vi "Utility Decode ID String.vi"(8 "error in (no error)":errorcluster, 10 "*IDN? Response":string, 11 "VISA resource name in":refnum<visa-resource-name>) -> (0 "error out":errorcluster, 2 "Unit Info":T1, 3 "VISA resource name out":refnum<visa-resource-name>)   [LabVIEW 2020, in "Berkeley Nucleonics 500 Series.lvlib"]
doc: "This VI decodes the response from an *IDN? query to return information about the unit It is private in scope."
uses:
  Berkeley Nucleonics 500 Series.lvlib
  Unit Info.ctl
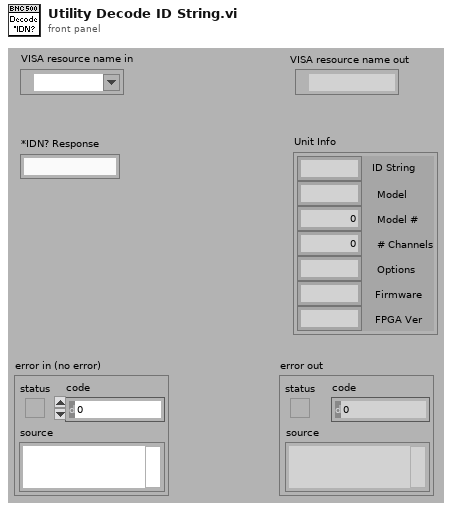
[diagram p1: front panel]
types:
  T1 = typedef "Berkeley Nucleonics 500 Series.lvlib/Unit Info.ctl" = cluster{"ID String":string, "Model":string, "Model #":i32, "# Channels":i32, "Options":string, "Firmware":string, "FPGA Ver":string}
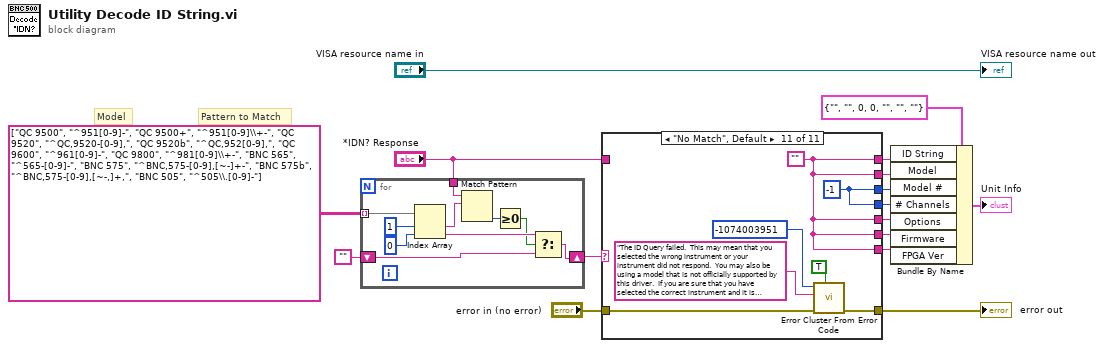
[diagram p0: block diagram]
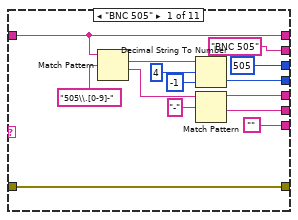
[diagram p2: hidden frame]
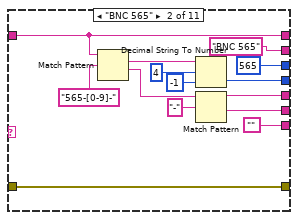
[diagram p3: hidden frame]
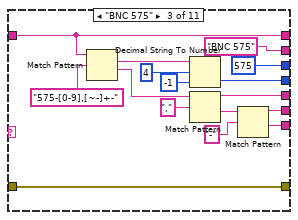
[diagram p4: hidden frame]
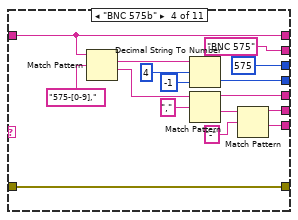
[diagram p5: hidden frame]
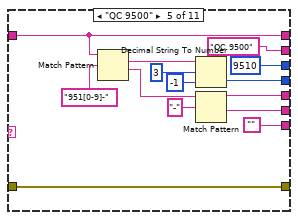
[diagram p6: hidden frame]
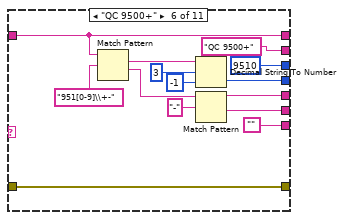
[diagram p7: hidden frame]
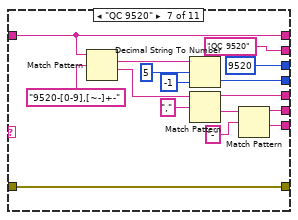
[diagram p8: hidden frame]
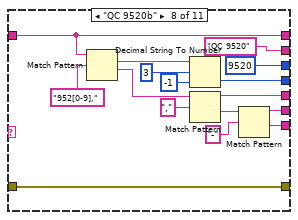
[diagram p9: hidden frame]
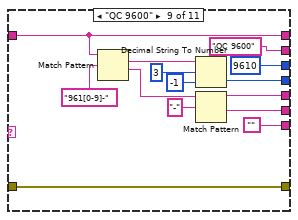
[diagram p10: hidden frame]
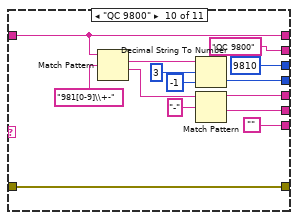
[diagram p11: hidden frame]
diagram:
  # "Pattern to Match"
  # "Model"
  n1 = for {
    tunnel: string[][] [["QC 9500", "^951[0-9]-"], ["QC 9500+", "^951[0-9]\\+-"], ["QC 9520", "^QC,9520-[0-9],"], ["QC 9520b", "^QC,952[0-9],"], ["QC 9600", "^961[0-9]-"], ["QC 9800", "^981[0-9]\\+-"], ["BNC 565", "^565-[0-9]-"], ["BNC 575", "^BNC,575-[0-9],[~-]+-"], ["BNC 575b", "^BNC,575-[0-9],[~-,]+,"], ["BNC 505", "^505\\.[0-9]-"]] ("appended array") -> [w24] mode=indexing
    tunnel: "*IDN? Response" -> [w25]
    shift-right: [w18] -> w6
    shift-left: "" -> [w19]
    n2 = Index Array(array=w24, index #1=1 ("index"), index #2=0 ("index")) -> (element #1=w23:string, element #2=w20:string)
    n3 = Match Pattern(string=w25, regular expression=w23) -> (offset past match=w26:i32)  [unwired: 1 in, 3 out]
    n4 = Greater Or Equal To 0?(x=w26) -> (x >= 0?=w17:bool)
    n5 = Select(t=w20, s=w17, f=w19) -> (s? t:f=w18:string)
  }
  n6 = case shown="\"No Match\", Default" w6 {
    tunnel: "*IDN? Response" -> [w38 w52 w68 w84 w98 w112 w128 w144 w158 w172 _]
    tunnel: [w38 w52 w68 w84 w98 w112 w128 w144 w158 w172 w180] -> w7
    tunnel: ["BNC 505" ("Model") "BNC 565" ("Model") "BNC 575" ("Model") "BNC 575" ("Model") "QC 9500" ("Model") "QC 9500+" ("Model") "QC 9520" ("Model") "QC 9520" ("Model") "QC 9600" ("Model") "QC 9800" ("Model") w180] -> w8
    tunnel: [505 ("Model #") 565 ("Model #") 575 ("Model #") 575 ("Model #") 9510 ("Model #") 9510 ("Model #") 9520 ("Model #") 9520 ("Model #") 9610 ("Model #") 9810 ("Model #") w181] -> w9
    tunnel: [w35 w49 w65 w81 w95 w109 w125 w141 w155 w169 w181] -> w10
    tunnel: [w31 w45 w63 w79 w91 w105 w123 w139 w151 w165 w180] -> w11
    tunnel: [w30 w44 w58 w74 w90 w104 w118 w134 w150 w164 w180] -> w12
    tunnel: ["" "" w57 w73 "" "" w117 w133 "" "" w180] -> w13
    tunnel: "error in (no error)" -> [w27 w41 w55 w71 w87 w101 w115 w131 w147 w161 w176]
    tunnel: [w27 w41 w55 w71 w87 w101 w115 w131 w147 w161 w175] -> w3
    frame "BNC 505" {
      n7 = Match Pattern(string=w38, regular expression="505\\.[0-9]-") -> (match substring=w34:string, after substring=w32:string)  [unwired: 1 in, 2 out]
      n8 = Decimal String To Number(string=w34, offset=4, default (0L)=-1) -> (number=w35:i32)  [unwired: 1 out]
      n9 = Match Pattern(string=w32, regular expression="-") -> (before substring=w31:string, after substring=w30:string)  [unwired: 1 in, 2 out]
    }
    frame "BNC 565" {
      n10 = Match Pattern(string=w52, regular expression="565-[0-9]-") -> (match substring=w48:string, after substring=w46:string)  [unwired: 1 in, 2 out]
      n11 = Decimal String To Number(string=w48, offset=4, default (0L)=-1) -> (number=w49:i32)  [unwired: 1 out]
      n12 = Match Pattern(string=w46, regular expression="-") -> (before substring=w45:string, after substring=w44:string)  [unwired: 1 in, 2 out]
    }
    frame "BNC 575" {
      n13 = Match Pattern(string=w68, regular expression="575-[0-9],[~-]+-") -> (match substring=w62:string, after substring=w61:string)  [unwired: 1 in, 2 out]
      n14 = Decimal String To Number(string=w62, offset=4, default (0L)=-1) -> (number=w65:i32)  [unwired: 1 out]
      n15 = Match Pattern(string=w61, regular expression=",") -> (before substring=w63:string, after substring=w59:string)  [unwired: 1 in, 2 out]
      n16 = Match Pattern(string=w59, regular expression="-") -> (before substring=w58:string, after substring=w57:string)  [unwired: 1 in, 2 out]
    }
    frame "BNC 575b" {
      n17 = Match Pattern(string=w84, regular expression="575-[0-9],") -> (match substring=w78:string, after substring=w77:string)  [unwired: 1 in, 2 out]
      n18 = Decimal String To Number(string=w78, offset=4, default (0L)=-1) -> (number=w81:i32)  [unwired: 1 out]
      n19 = Match Pattern(string=w77, regular expression=",") -> (before substring=w79:string, after substring=w75:string)  [unwired: 1 in, 2 out]
      n20 = Match Pattern(string=w75, regular expression="-") -> (before substring=w74:string, after substring=w73:string)  [unwired: 1 in, 2 out]
    }
    frame "QC 9500" {
      n21 = Match Pattern(string=w98, regular expression="951[0-9]-") -> (match substring=w94:string, after substring=w92:string)  [unwired: 1 in, 2 out]
      n22 = Decimal String To Number(string=w94, offset=3, default (0L)=-1) -> (number=w95:i32)  [unwired: 1 out]
      n23 = Match Pattern(string=w92, regular expression="-") -> (before substring=w91:string, after substring=w90:string)  [unwired: 1 in, 2 out]
    }
    frame "QC 9500+" {
      n24 = Match Pattern(string=w112, regular expression="951[0-9]\\+-") -> (match substring=w108:string, after substring=w106:string)  [unwired: 1 in, 2 out]
      n25 = Decimal String To Number(string=w108, offset=3, default (0L)=-1) -> (number=w109:i32)  [unwired: 1 out]
      n26 = Match Pattern(string=w106, regular expression="-") -> (before substring=w105:string, after substring=w104:string)  [unwired: 1 in, 2 out]
    }
    frame "QC 9520" {
      n27 = Match Pattern(string=w128, regular expression="9520-[0-9],[~-]+-") -> (match substring=w122:string, after substring=w121:string)  [unwired: 1 in, 2 out]
      n28 = Decimal String To Number(string=w122, offset=5, default (0L)=-1) -> (number=w125:i32)  [unwired: 1 out]
      n29 = Match Pattern(string=w121, regular expression=",") -> (before substring=w123:string, after substring=w119:string)  [unwired: 1 in, 2 out]
      n30 = Match Pattern(string=w119, regular expression="-") -> (before substring=w118:string, after substring=w117:string)  [unwired: 1 in, 2 out]
    }
    frame "QC 9520b" {
      n31 = Match Pattern(string=w144, regular expression="952[0-9],") -> (match substring=w138:string, after substring=w137:string)  [unwired: 1 in, 2 out]
      n32 = Decimal String To Number(string=w138, offset=3, default (0L)=-1) -> (number=w141:i32)  [unwired: 1 out]
      n33 = Match Pattern(string=w137, regular expression=",") -> (before substring=w139:string, after substring=w135:string)  [unwired: 1 in, 2 out]
      n34 = Match Pattern(string=w135, regular expression="-") -> (before substring=w134:string, after substring=w133:string)  [unwired: 1 in, 2 out]
    }
    frame "QC 9600" {
      n35 = Match Pattern(string=w158, regular expression="961[0-9]-") -> (match substring=w154:string, after substring=w152:string)  [unwired: 1 in, 2 out]
      n36 = Decimal String To Number(string=w154, offset=3, default (0L)=-1) -> (number=w155:i32)  [unwired: 1 out]
      n37 = Match Pattern(string=w152, regular expression="-") -> (before substring=w151:string, after substring=w150:string)  [unwired: 1 in, 2 out]
    }
    frame "QC 9800" {
      n38 = Match Pattern(string=w172, regular expression="981[0-9]\\+-") -> (match substring=w168:string, after substring=w166:string)  [unwired: 1 in, 2 out]
      n39 = Decimal String To Number(string=w168, offset=3, default (0L)=-1) -> (number=w169:i32)  [unwired: 1 out]
      n40 = Match Pattern(string=w166, regular expression="-") -> (before substring=w165:string, after substring=w164:string)  [unwired: 1 in, 2 out]
    }
    frame "No Match", Default {
      w181 = -1 ("Model #")
      w180 = ""
      n41 = call <vilib>:"Error Cluster From Error Code.vi"("show call chain? (False)"=TRUE, "error in (no error)"=w176, "error message (\"\")"="The ID Query failed.  This may mean that you selected the wrong instrument or your instrument did not respond.  You may also be using a model that is not officially supported by this driver.  If you are sure that you have selected the correct instrument and it is responding, try disabling the ID Query." ("Source (VI Name)"), "error code (0)"=-1074003951 ("Code")) -> ("error out"=w175:errorcluster)  [unwired: 5 in]
    }
  }
  "error out" <- w3
  n42 = Bundle By Name(cluster=T1 {"ID String"="", "Model"="", "Model #"=0, "# Channels"=0, "Options"="", "Firmware"="", "FPGA Ver"=""} ("Unit Info"), "ID String"=w7, "Model"=w8, "Model #"=w9, "# Channels"=w10, "Options"=w11, "Firmware"=w12, "FPGA Ver"=w13) -> (→"Unit Info":T1)
  "VISA resource name out" <- "VISA resource name in"
